vi "Build Low Priority Data Field.vi"(6 "Group":i32, 7 "Virtual Memory Unit in":refnum<class "Virtual Memory Unit.lvclass">, 8 "error in (no error)":errorcluster, 10 "Starting Address":u16 format="%04x", 11 "Major Frame in":refnum<class "Major Frame.lvclass">) -> (0 "error out":errorcluster, 2 "Next Available Address":u16 format="%04x", 3 "Major Frame out":refnum<class "Major Frame.lvclass">, 5 "Virtual Memory Unit out":refnum<class "Virtual Memory Unit.lvclass">)   [LabVIEW 2020, in "BCI-1553 API.lvlib" / "Major Frame.lvclass"]
doc: "Puts easily-identifiable data into the LP Async Data Field.\n\nThis is exclusively for debug and validation. The async send method will overwrite all the relevant data words."
uses:
  Major Frame.lvclass
  Dependencies/Virtual Memory Unit/Virtual Memory Unit.lvclass
  Major Frame.lvclass/Major Frame.ctl
  BCI-1553 API.lvlib
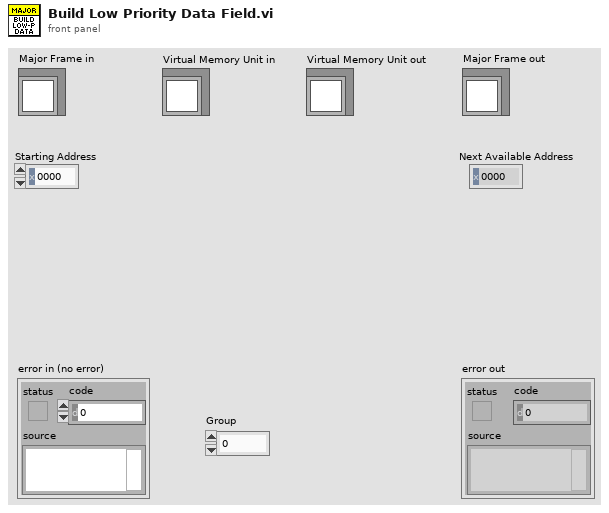
[diagram p1: front panel]
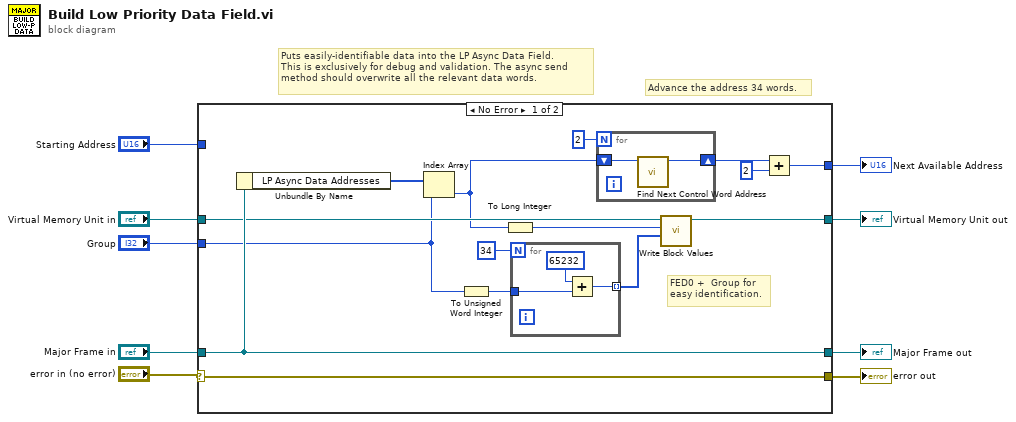
[diagram p0: block diagram]
diagram:
  # "Advance the address 34 words."
  # "Puts easily-identifiable data into the LP Async Data Field.\nThis is exclusively for debug and validation. The async send\nmethod should overwrite all the relevant data words."
  n1 = case shown="No Error" "error in (no error)" {
    selector: "error in (no error)" -> [w23 w31]
    tunnel: [w23 w31] -> w1
    tunnel: [w22 w30] -> w2
    tunnel: "Major Frame in" -> [w22 w30]
    tunnel: "Virtual Memory Unit in" -> [w17 _]
    tunnel: [w16 _] -> w4
    tunnel: "Group" -> [w11 _]
    tunnel: [w18 _] -> w3
    tunnel: "Starting Address" -> [_ _]
    frame No Error {
      # "FED0 +  Group for\neasy identification."
      n2 = Unbundle By Name(w22) -> ("LP Async Data Addresses"=w24:u16[])
      n3 = Index Array(array=w24, index=w11) -> (element=w14:u16)
      n4 = To Unsigned Word Integer(number=w11) -> (unsigned 16bit integer=w10:u16)
      n5 = To Long Integer(number=w14) -> (32bit integer=w15:i32)
      n6 = for {
        N: 34 ("dimension size") -> [_]
        tunnel: [w25] -> w12 mode=indexing
        tunnel: w10 -> [w27]
        n7 = Add(x=u16 65232 ("element"), y=w27) -> (x+y=w25:u16)
      }
      n8 = for {
        N: 2 -> [_]
        shift-right: [w28] -> w20
        shift-left: w14 -> [w29]
        n9 = call "Find Next Control Word Address.vi"("Starting Address"=w29) -> ("0xHHHX Address"=w28:u16)  [unwired: 10 in]
      }
      n10 = call "Write Block Values.vi"("Write Block"=w12, "Start Index"=w15, "Virtual Memory Unit in"=w17) -> ("Virtual Memory Unit out"=w16:refnum<class "Virtual Memory Unit.lvclass">)  [unwired: 7 in, 1 out]
      n11 = Add(x=w20, y=u16 2) -> (x+y=w18:u16)
    }
    frame Error {
    }
  }
  "error out" <- w1
  "Major Frame out" <- w2
  "Next Available Address" <- w3
  "Virtual Memory Unit out" <- w4
